vi "Update Plugin Metadata by Reference.vi"(8 "error in (no error)":errorcluster, 10 "plugin_metadata":T1, 11 "Metadata":refnum<vi>) -> (0 "error out":errorcluster)   [LabVIEW 2021, in "CIF_Manager_UI.lvclass"]
uses:
  CIF_Manager_UI.lvclass
  <vilib>/CIF Foundation/CIF Core/CIFPluginManager/gRPC/CIF_Manager_client/RPC Messages/cif_management_common_PluginMetadata.ctl
  <vilib>/CIF Foundation/CIF Core/CIFPluginManager/gRPC/CIF_Manager_client/CIF_Manager_client.lvlib
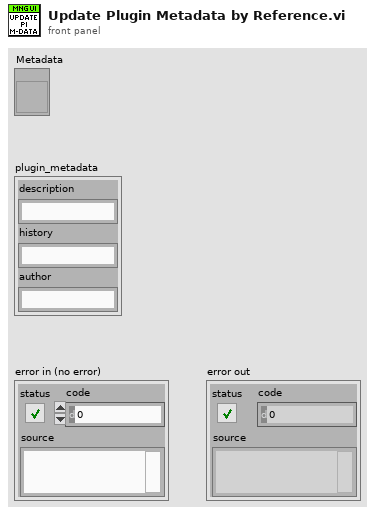
[diagram p1: front panel]
types:
  T1 = typedef "CIF_Manager_client.lvlib/cif_management_common_PluginMetadata.ctl" = cluster{"description":string, "history":string, "author":string}
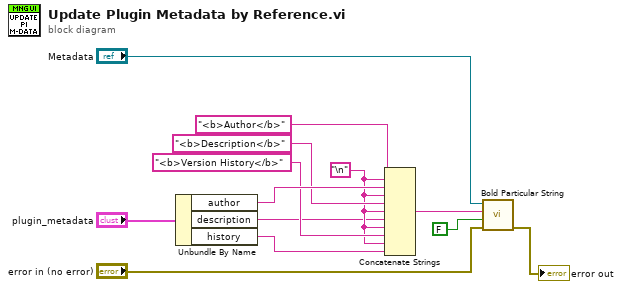
[diagram p0: block diagram]
diagram:
  w8 = "\n"
  n1 = Unbundle By Name("plugin_metadata") -> ("author"=w11:string, "description"=w7:string, "history"=w6:string)
  n2 = Concatenate Strings("<b>Author</b>" ("string"), w8, w11, w8, "<b>Description</b>" ("string"), w8, w7, w8, "<b>Version History</b>" ("string"), w8, w6) -> (w5:string)
  n3 = call <vilib>:"Bold Particular String.vi"("error in (no error)"="error in (no error)", "resize string? (TRUE)"=FALSE, "text to display"=w5, "string refnum"="Metadata") -> ("error out"=→"error out":errorcluster)  [unwired: 6 in, 1 out]
